vi "init_laser.vi"(7 "Pulsed":bool, 8 "Voltage limits":T2={"maximum value"=5.0, "minimum value"=0.0} {"minimum value" format="%#_13g"; "maximum value" format="%#_13g"}, 9 "channel parameters":T1={"voltage"=0.0, "frequency"=0.0, "duty cycle"=0.0, "sample rate"=1000.0}, 10 "name to assign":string="laser", 11 "physical channels":tag) -> (0 "error out":errorcluster, 3 "task out":refnum<k21>)   [LabVIEW 2025]
uses:
  channel parameters cluster.ctl
  <vilib>/DAQmx/write.llb/DAQmx Write (Analog DBL 1Chan 1Samp).vi
  <vilib>/DAQmx/write.llb/DAQmx Write (Analog Wfm 1Chan NSamp).vi
  <vilib>/DAQmx/create/channels.llb/DAQmx Create Channel (AO-Voltage-Basic).vi
  <vilib>/DAQmx/configure/timing.llb/DAQmx Timing (Sample Clock).vi
  <vilib>/DAQmx/miscellaneous.llb/DAQmx Fill In Error Info.vi
  <resource>/objmgr/daqmx.rc
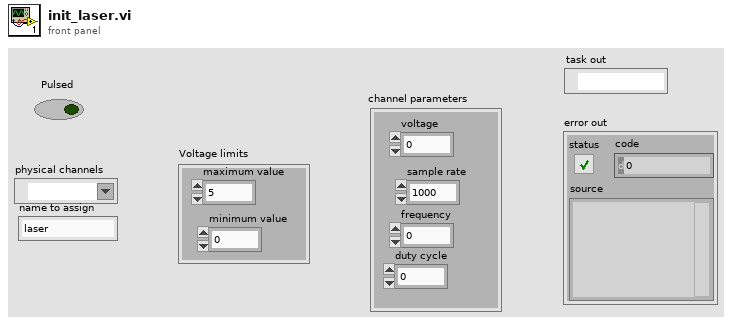
[diagram p1: front panel]
types:
  T1 = typedef "channel parameters cluster.ctl" = cluster{"voltage":dbl, "frequency":dbl, "duty cycle":dbl, "sample rate":dbl}
  T2 = cluster{"maximum value":dbl, "minimum value":dbl}
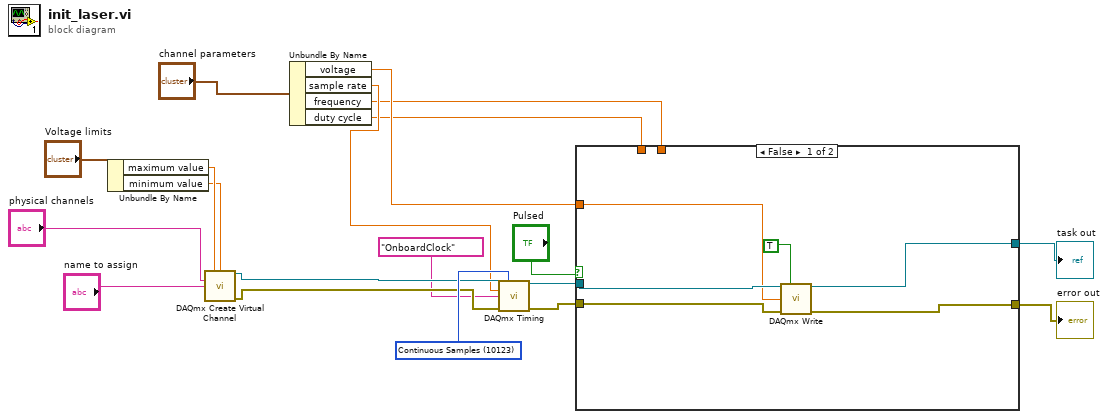
[diagram p0: block diagram]
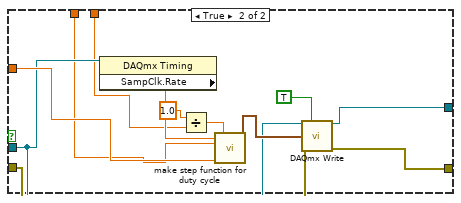
[diagram p2: hidden frame]
diagram:
  w17 = 10123 items=["Finite Samples"=10178, "Continuous Samples"=10123, "Hardware Timed Single Point"=12522] ("SampQuant.SampMode")
  n1 = Unbundle By Name("Voltage limits") -> ("maximum value"=w12:dbl, "minimum value"=w11:dbl)
  n2 = call-poly <vilib>:"DAQmx Create Virtual Channel.vi"("maximum value"=w12, "minimum value"=w11, "physical channels"="physical channels", "name to assign"="name to assign") -> ("task out"=w15:refnum<k21>, "error out"=w16:errorcluster)  [unwired: 10 in]
  n3 = Unbundle By Name("channel parameters") -> ("voltage"=w4:dbl, "sample rate"=w3:dbl, "frequency"=w1:dbl, "duty cycle"=w2:dbl)
  n4 = call-poly <vilib>:"DAQmx Timing.vi"("task/channels in"=w15, "sample mode"=w17, "rate"=w3, "source"=tag "OnboardClock", "error in"=w16) -> ("task out"=w9:refnum<k21>, "error out"=w8:errorcluster)  [unwired: 9 in]
  n5 = case shown="False" "Pulsed" {
    tunnel: w9 -> [w25 w31]
    tunnel: w8 -> [w24 w30]
    tunnel: [w23 w34] -> w7
    tunnel: [w22 w33] -> w6
    tunnel: w4 -> [w21 w32]
    tunnel: w2 -> [_ w28]
    tunnel: w1 -> [_ w27]
    frame False {
      n6 = call-poly <vilib>:"DAQmx Write.vi"("task/channels in"=w25, "auto start"=TRUE, "data"=w21, "error in"=w24) -> ("task out"=w22:refnum<k21>, "error out"=w23:errorcluster)  [unwired: 9 in, 1 out]
    }
    frame True {
      n7 = property class="DAQmx Timing"(reference=w31) -> ("SampClk.Rate"=w36:dbl)  [unwired: 1 in, 2 out]
      n8 = Divide(x=1.0, y=w27) -> (x/y=w29:dbl)
      n9 = call "make step function for duty cycle.vi"("amplitude"=w32, "period"=w29, "duty cycle"=w28, "sample rate"=w36) -> ("Waveform out"=w35:waveform(dbl))  [unwired: 7 in]
      n10 = call-poly <vilib>:"DAQmx Write.vi"("task/channels in"=w31, "auto start"=TRUE, "data"=w35, "error in"=w30) -> ("task out"=w33:refnum<k21>, "error out"=w34:errorcluster)  [unwired: 9 in, 1 out]
    }
  }
  "error out" <- w7
  "task out" <- w6
